vi "Asylum_SoftReset.vi"(8 "error in (no error)":errorcluster, 11 "Application":refnum<k7>) -> (0 "error out":errorcluster, 3 "Application":refnum<k7>)   [LabVIEW 2019]
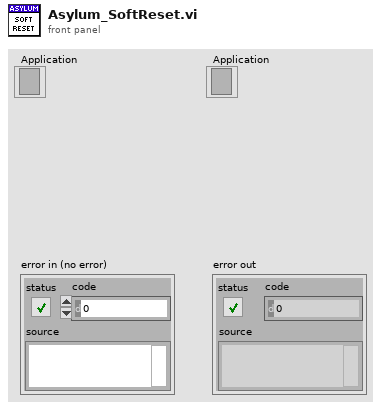
[diagram p1: front panel]
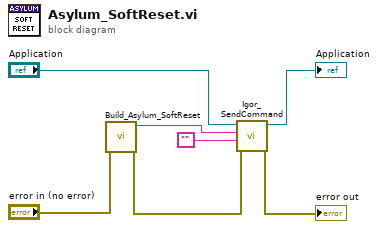
[diagram p0: block diagram]
diagram:
  n1 = call "Build_Asylum_SoftReset.vi"("error in (no error)"="error in (no error)") -> ("error out"=w7:errorcluster, "Command"=w5:string)  [unwired: 9 in]
  n2 = call <userlib>:"Igor_SendCommand.vi"("error in (no error)"=w7, "Format"="", "command"=w5, "Application In"="Application") -> ("error out"=→"error out":errorcluster, "Application Out"=→"Application":refnum<k7>)  [unwired: 4 in, 2 out]
